vi "xy波形图.vi"() -> ()   [LabVIEW 2010]
uses:
  <vilib>/Analysis/NI_AALBase.lvlib
panel:
  out "XY图":cluster{cluster{dbl, dbl}[]}[](graph)
  out "XY图":T1(graph)
  out "XY图":cluster{dbl, dbl}[](graph)
  out "XY图":T2(graph)
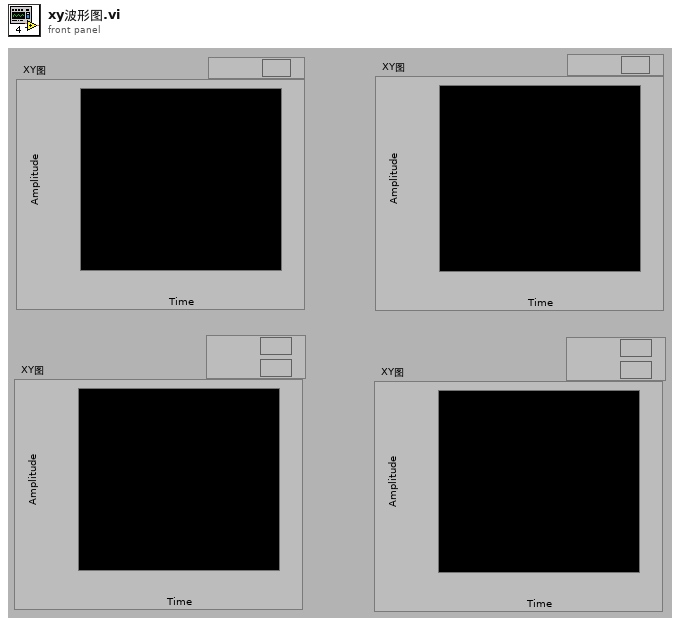
[diagram p1: front panel]
types:
  T1 = cluster{"Sinusoidal Pattern":dbl[], "Sinusoidal Pattern":dbl[]}[]
  T2 = cluster{"Sinusoidal Pattern":dbl[], "Sinusoidal Pattern":dbl[]}
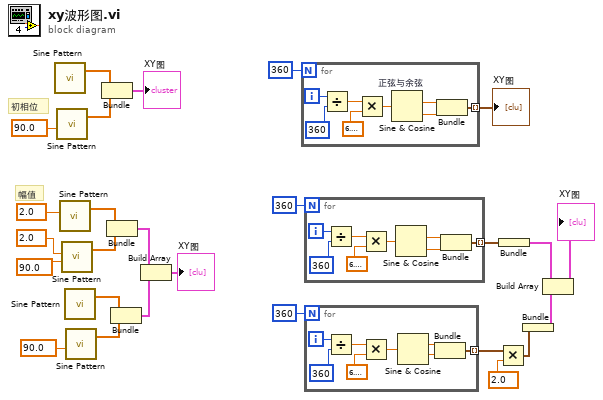
[diagram p0: block diagram]
diagram:
  # "幅值"
  # "初相位"
  n1 = call <vilib>:"Sine Pattern.vi"() -> ("Sinusoidal Pattern"=w25:dbl[])  [unwired: 4 in, 1 out]
  n2 = call <vilib>:"Sine Pattern.vi"("phase(degrees)"=90.0) -> ("Sinusoidal Pattern"=w24:dbl[])  [unwired: 3 in, 1 out]
  n3 = call <vilib>:"Sine Pattern.vi"("amplitude"=2.0) -> ("Sinusoidal Pattern"=w19:dbl[])  [unwired: 3 in, 1 out]
  n4 = call <vilib>:"Sine Pattern.vi"("phase(degrees)"=90.0, "amplitude"=2.0) -> ("Sinusoidal Pattern"=w20:dbl[])  [unwired: 2 in, 1 out]
  n5 = call <vilib>:"Sine Pattern.vi"() -> ("Sinusoidal Pattern"=w16:dbl[])  [unwired: 4 in, 1 out]
  n6 = call <vilib>:"Sine Pattern.vi"("phase(degrees)"=90.0) -> ("Sinusoidal Pattern"=w15:dbl[])  [unwired: 3 in, 1 out]
  n7 = Bundle("Sinusoidal Pattern"=w25, "Sinusoidal Pattern"=w24) -> (→"XY图":T2)  [unwired: 1 in]
  n8 = Bundle("Sinusoidal Pattern"=w19, "Sinusoidal Pattern"=w20) -> (w14:T2)  [unwired: 1 in]
  n9 = Bundle("Sinusoidal Pattern"=w16, "Sinusoidal Pattern"=w15) -> (w13:T2)  [unwired: 1 in]
  n10 = Build Array(w14, w13) -> (→"XY图":T1)
  n11 = for {
    N: 360 -> [_]
    tunnel: [w33] -> w21 mode=indexing
    i -> [w30]
    n12 = Divide(x=w30, y=360) -> (x/y=w28:dbl)
    n13 = Multiply(x=w28, y=6.283185307179586) -> (x*y=w29:dbl)
    n14 = Sine & Cosine "正弦与余弦"(0:w29) -> (1:w34:dbl, 2:w27:dbl)
    n15 = Bundle(w34, w27) -> (w33:cluster{dbl, dbl})  [unwired: 1 in]
  }
  "XY图" <- w21
  n16 = for {
    N: 360 -> [_]
    tunnel: [w41] -> w5 mode=indexing
    i -> [w38]
    n17 = Divide(x=w38, y=360) -> (x/y=w36:dbl)
    n18 = Multiply(x=w36, y=6.283185307179586) -> (x*y=w37:dbl)
    n19 = Sine & Cosine(0:w37) -> (1:w42:dbl, 2:w35:dbl)
    n20 = Bundle(w42, w35) -> (w41:cluster{dbl, dbl})  [unwired: 1 in]
  }
  n21 = for {
    N: 360 -> [_]
    tunnel: [w50] -> w6 mode=indexing
    i -> [w47]
    n22 = Divide(x=w47, y=360) -> (x/y=w45:dbl)
    n23 = Multiply(x=w45, y=6.283185307179586) -> (x*y=w46:dbl)
    n24 = Sine & Cosine(0:w46) -> (1:w44:dbl, 2:w43:dbl)
    n25 = Bundle(w44, w43) -> (w50:cluster{dbl, dbl})  [unwired: 1 in]
  }
  n26 = Multiply(x=w6, y=2.0) -> (x*y=w3:cluster{dbl, dbl}[])
  n27 = Bundle(w5) -> (w4:cluster{cluster{dbl, dbl}[]})  [unwired: 1 in]
  n28 = Bundle(w3) -> (w2:cluster{cluster{dbl, dbl}[]})  [unwired: 1 in]
  n29 = Build Array(w4, w2) -> (→"XY图":cluster{cluster{dbl, dbl}[]}[])
